vi "Determine Warnings-SUBVI.vi"(8 "error in (no error)":errorcluster, 9 "Min Temp":dbl, 10 "Max Temp":dbl, 11 "Current Temp":dbl) -> (0 "error out":errorcluster, 1 "Warning?":bool, 2 "Warning Text":string)   [LabVIEW 2014]
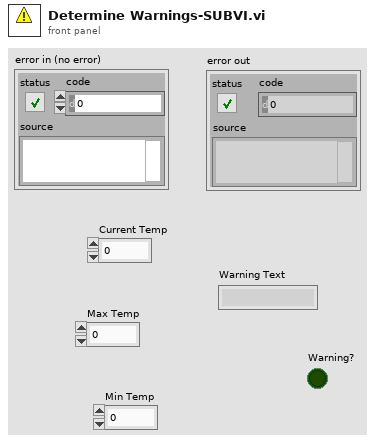
[diagram p1: front panel]
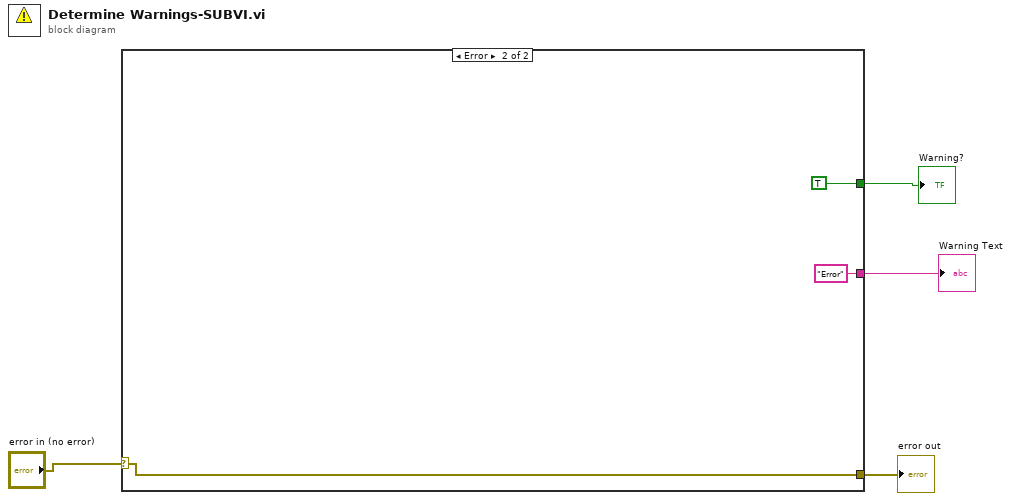
[diagram p0: block diagram]
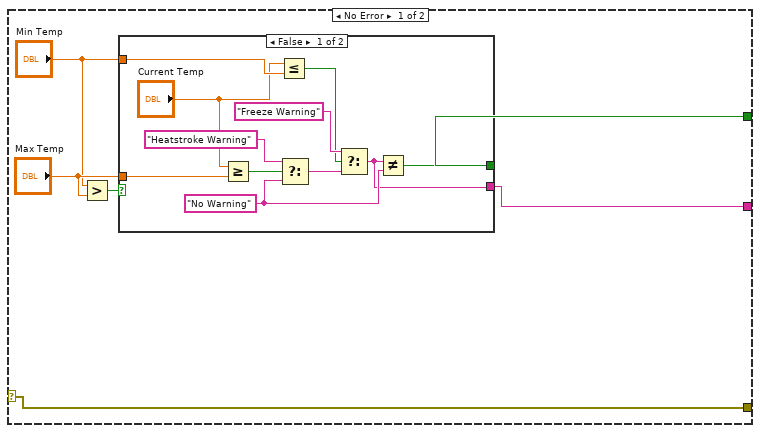
[diagram p2: hidden frame]
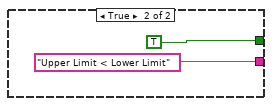
[diagram p3: hidden frame]
diagram:
  n1 = case shown="Error" "error in (no error)" {
    selector: "error in (no error)" -> [w5 w24]
    tunnel: [w7 "Error"] -> w4
    tunnel: [w6 TRUE] -> w3
    tunnel: [w5 w24] -> w1
    frame No Error {
      n2 = Greater?(x="Min Temp", y="Max Temp") -> (0:w8:bool)
      n3 = case shown="False" w8 {
        tunnel: "Min Temp" -> [w21 _]
        tunnel: "Max Temp" -> [w19 _]
        tunnel: [w12 TRUE] -> w6
        tunnel: [w11 "Upper Limit < Lower Limit"] -> w7
        frame False {
          w18 = "No Warning"
          n4 = Greater Or Equal?(x="Current Temp", y=w19) -> (x >= y?=w14:bool)
          n5 = Less Or Equal?(x="Current Temp", y=w21) -> (x <= y?=w13:bool)
          n6 = Select(t="Heatstroke Warning", s=w14, f=w18) -> (s? t:f=w17:string)
          n7 = Select(t="Freeze Warning", s=w13, f=w17) -> (s? t:f=w11:string)
          n8 = Not Equal?(x=w11, y=w18) -> (x != y?=w12:bool)
        }
        frame True {
        }
      }
    }
    frame Error {
    }
  }
  "error out" <- w1
  "Warning?" <- w3
  "Warning Text" <- w4
